vi "Write 2D Error Bar Property Array.vi"(8 "error in (no error)":errorcluster, 10 "2D Error Bar Property Array":T1, 11 "2D Error Bar.lvclass in":refnum<class "2D Error Bar.lvclass">) -> (0 "error out":errorcluster, 3 "2D Error Bar.lvclass out":refnum<class "2D Error Bar.lvclass">)   [LabVIEW 2017, in "2D Error Bar.lvclass"]
uses:
  <vilib>/Math Plots/2D Math Plots/2D Error Bar/2D Error Bar/2D Error Bar.lvclass
  <vilib>/Math Plots/2D Math Plots/2D Error Bar/2D Error Bar/Typedef/2D Error Bar Property Array.ctl
  <vilib>/Math Plots/2D Math Plots/2D Error Bar/2D Error Bar/Typedef/2D Error Bar Property.ctl
  <vilib>/Math Plots/2D Math Plots/2D Error Bar/2D Error Bar/2D Error Bar.lvclass/2D Error Bar.ctl
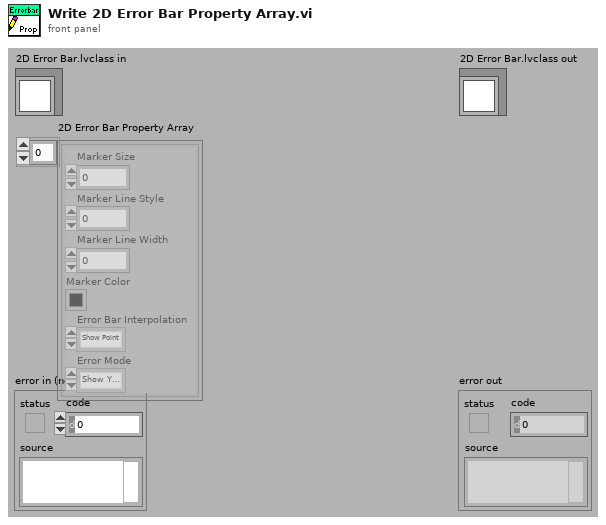
[diagram p1: front panel]
types:
  T1 = typedef "2D Error Bar.lvclass/2D Error Bar Property Array.ctl" = T2[]
  T2 = typedef "2D Error Bar.lvclass/2D Error Bar Property.ctl" = cluster{"Marker Size":dbl, "Marker Line Style":u8, "Marker Line Width":u8, "Marker Color":u32, "Error Bar Interpolation":enum16{"Show Point", "Show Line", "Show Bar"}, "Error Mode":enum16{"Show Y Error", "Show X Error", "Show Both Error"}}
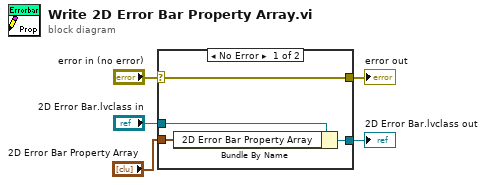
[diagram p0: block diagram]
diagram:
  n1 = case shown="No Error" "error in (no error)" {
    selector: "error in (no error)" -> [w9 w10]
    tunnel: [w9 w10] -> w4
    tunnel: [w7 w11] -> w2
    tunnel: "2D Error Bar.lvclass in" -> [w8 w11]
    tunnel: "2D Error Bar Property Array" -> [w6 _]
    frame No Error {
      n2 = Bundle By Name(cluster=w8, "2D Error Bar Property Array"=w6) -> (w7:refnum<class "2D Error Bar.lvclass">)
    }
    frame Error {
    }
  }
  "error out" <- w4
  "2D Error Bar.lvclass out" <- w2
